vi "unpackAutonArray.vi"(9 "all rows":dbl[][](array[numeric])) -> (0 "Distance/time":dbl[](array[numeric]), 1 "Heading/Shoot angle":dbl[](array[numeric]), 2 "Power/Arm":dbl[](array[numeric]), 3 "Primitive":i16[](array[numeric]), 4 "Misc":dbl[](array[numeric]))   [LabVIEW 2013]
doc: "Use this VI to separate the autonomous array data into individual arrays. First array is Primitive ID, second is heading, etc."
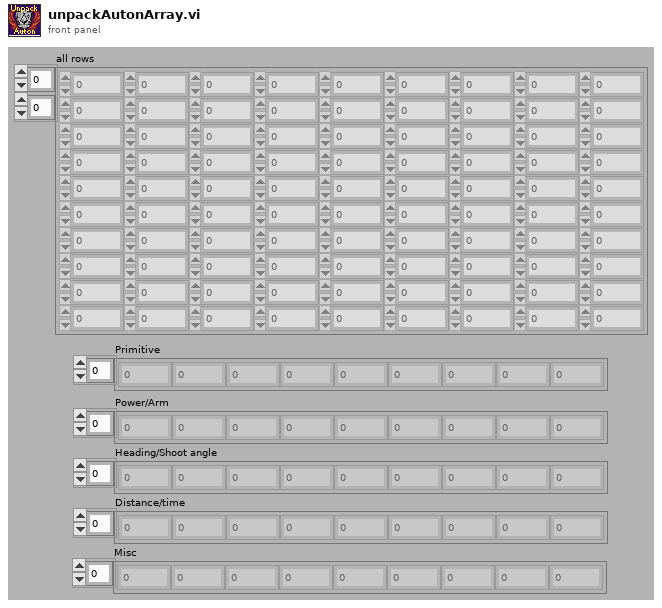
[diagram p1: front panel]
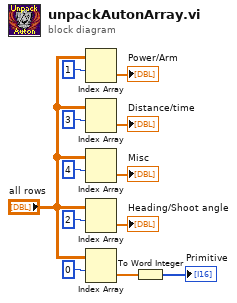
[diagram p0: block diagram]
diagram:
  n1 = Index Array(array="all rows", index (row)=1) -> (element=→"Power/Arm":dbl[])  [unwired: 1 in]
  n2 = Index Array(array="all rows", index (row)=3) -> (element=→"Distance/time":dbl[])  [unwired: 1 in]
  n3 = Index Array(array="all rows", index (row)=4) -> (element=→"Misc":dbl[])  [unwired: 1 in]
  n4 = Index Array(array="all rows", index (row)=2) -> (element=→"Heading/Shoot angle":dbl[])  [unwired: 1 in]
  n5 = Index Array(array="all rows", index (row)=0) -> (element=w7:dbl[])  [unwired: 1 in]
  n6 = To Word Integer(number=w7) -> (16bit integer=→"Primitive":i16[])
